vi "Input_Shared_Variable.vi"() -> (0 "Machine Out":string, 1 "Shared Variable Out":refnum<k21>, 2 "Type out":string)   [LabVIEW 2016]
panel:
  in  "Machine":string
  in  "Type":string
  in  "Continue":bool
  in  "New Variable":refnum<k21>
  # "Input your new variable here:"
  # "What does the variable track?"
  # "What machine is the variable for?"
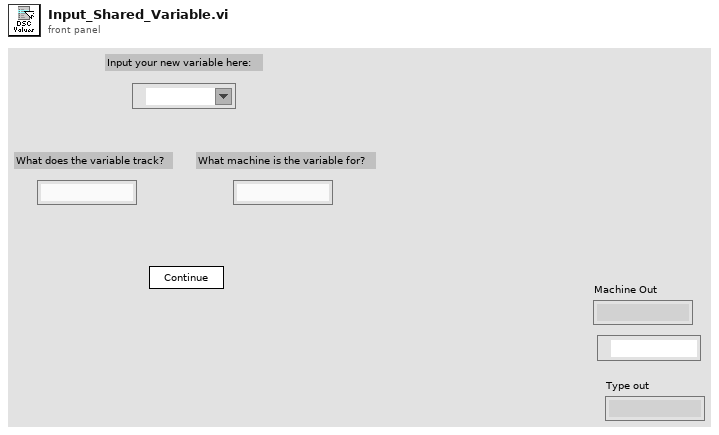
[diagram p1: front panel]
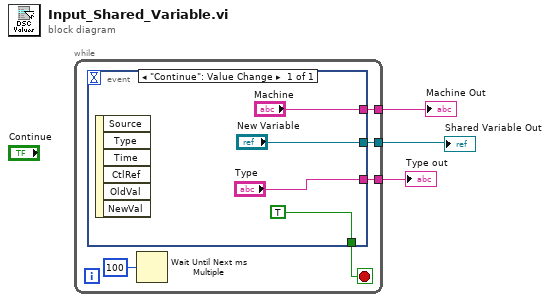
[diagram p0: block diagram]
diagram:
  n1 = while {
    tunnel: [w6] -> w3
    tunnel: [w5] -> w2
    tunnel: [w4] -> w1
    stop <- w8 stop-if-true
    n2 = event shown="[0] \"Continue\": Value Change" {
      selector: _ -> [_]
      dyn-events: _ -> [_]
      timeout: _ -> [_]
      tunnel: [TRUE] -> w8
      tunnel: ["New Variable"] -> w6
      tunnel: ["Type"] -> w5
      tunnel: ["Machine"] -> w4
      event "Continue": Value Change {
        n3 = event-data() -> ()  [unwired: 1 in, 6 out]
      }
    }
    n4 = Wait Until Next ms Multiple(millisecond multiple=u32 100) -> ()  [unwired: 1 out]
  }
  "Shared Variable Out" <- w3
  "Type out" <- w2
  "Machine Out" <- w1
